vi "from string array.vi"(8 "error in (no error)":errorcluster, 9 "String Array":string[][](array[string]), 10 "version":string, 11 "module configuration in":refnum<class "tag select module configuration.lvclass">) -> (0 "error out":errorcluster, 3 "module configuration out":refnum<class "tag select module configuration.lvclass">)   [LabVIEW 2015, in "tag select module configuration.lvclass"]
uses:
  tag select module configuration.lvclass
  tag select configuration.ctl
  <vilib>/NI/Tag Bus/tag/Data Type.ctl
  <vilib>/NI/Tag Bus Module Framework/channel/TBM channel.lvclass
  <vilib>/NI/Tag Bus Module Framework/channel/channel classification.ctl
  tag select module configuration.lvclass/tag select module configuration.ctl
  Write tag select.vi
  <vilib>/NI/Tag Bus/tag/tag descriptor.lvclass
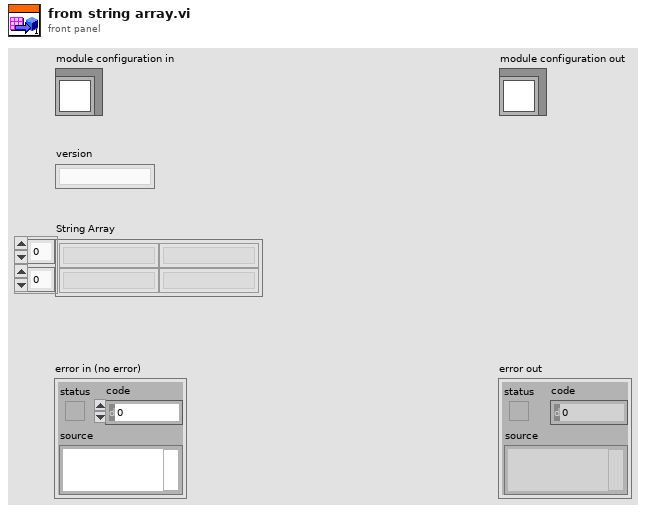
[diagram p1: front panel]
types:
  T1 = typedef "tag bus.lvlib/tag descriptor.lvclass/Data Type.ctl" = enum16{"Double", "Single", "I64", "I32", "I16", "I8", "U64", "U32", "U16", "U8", "Boolean", "String", "Array of Double", "Array of Single", "Array of I64", "Array of I32", "Array of I16", "Array of I8", "Array of U64", "Array of U32", "Array of U16", "Array of U8", "Array of Boolean", "Array of String"}
  T2 = typedef "TBM channel.lvclass/channel classification.ctl" = enum16{"input data", "output data", "processing parameter", "processing result"}
  T3 = typedef "tag select module configuration.lvclass/tag select configuration.ctl" = cluster{"tag select name":string, "data type":T1, "output":refnum<class "TBM channel.lvclass">, "select":refnum<class "TBM channel.lvclass">, "input channels":refnum<class "TBM channel.lvclass">[]}
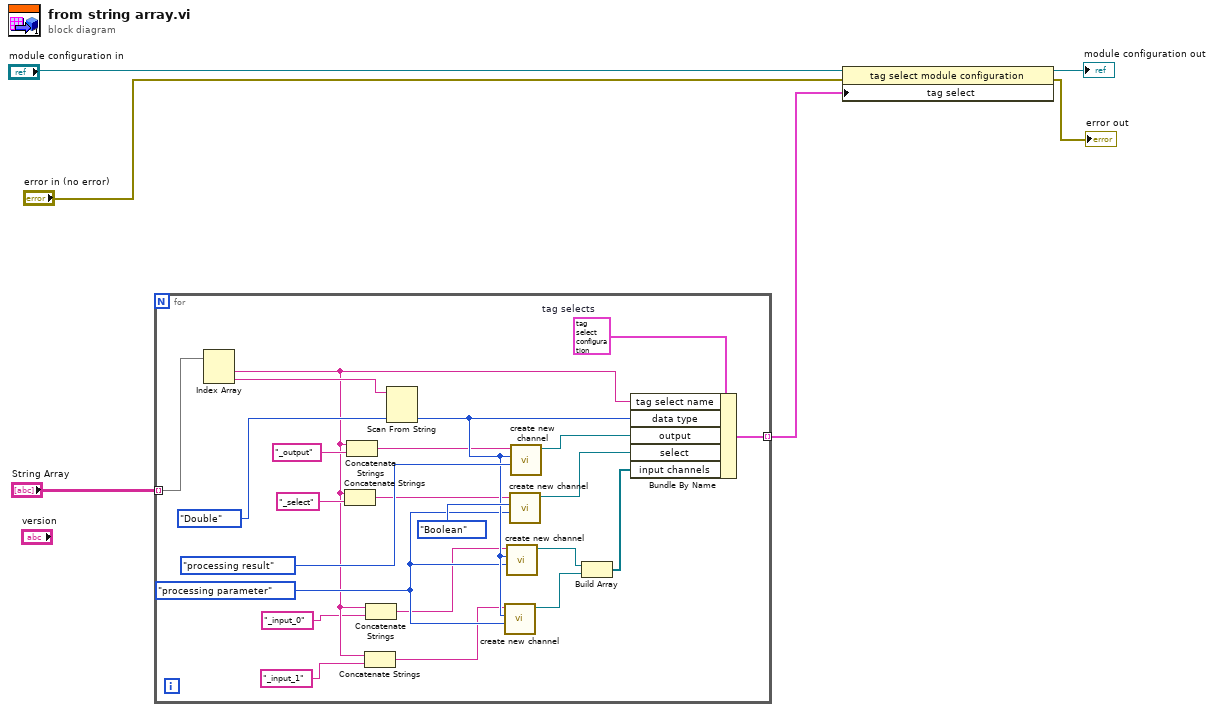
[diagram p0: block diagram]
diagram:
  n1 = for {
    tunnel: "String Array" -> [w28] mode=indexing
    tunnel: [w17] -> w1 mode=indexing
    w16 = channel_classification."processing parameter" ("channel classification")
    w29 = T3 {"tag select name"="", "data type"=enum."Double", "output"=refnum, "select"=refnum, "input channels"=[]}  # tag selects
    n2 = Index Array "Index Array"(array=w28) -> (element #1=w9:string, element #2=w27:string)  [unwired: 2 in]
    n3 = Concatenate Strings(w9, "_select" ("string")) -> (w13:string)
    n4 = Concatenate Strings(w9, "_output" ("string")) -> (w14:string)
    n5 = Concatenate Strings(w9, "_input_1" ("string")) -> (w10:string)
    n6 = Concatenate Strings(w9, "_input_0" ("string")) -> (w11:string)
    n7 = Scan From String(input string=w27, default 1=Data_Type."Double" ("data type")) -> (output 1=w21:T1)  [unwired: 3 in, 3 out]
    n8 = call <vilib>:"create new channel.vi"("channel classification"=w16, "data type"=w21, "channel name"=w10) -> ("channel"=w20:refnum<class "TBM channel.lvclass">)  [unwired: 8 in]
    n9 = call <vilib>:"create new channel.vi"("channel classification"=w16, "data type"=w21, "channel name"=w11) -> ("channel"=w19:refnum<class "TBM channel.lvclass">)  [unwired: 8 in]
    n10 = call <vilib>:"create new channel.vi"("channel classification"=w16, "data type"=Data_Type."Boolean", "channel name"=w13) -> ("channel"=w23:refnum<class "TBM channel.lvclass">)  [unwired: 8 in]
    n11 = call <vilib>:"create new channel.vi"("channel classification"=channel_classification."processing result", "data type"=w21, "channel name"=w14) -> ("channel"=w25:refnum<class "TBM channel.lvclass">)  [unwired: 8 in]
    n12 = Build Array(w19, w20) -> (w18:refnum<class "TBM channel.lvclass">[])
    n13 = Bundle By Name(cluster=w29, "tag select name"=w9, "data type"=w21, "output"=w25, "select"=w23, "input channels"=w18) -> (w17:T3)
  }
  n14 = property class="tag select module configuration"(reference="module configuration in", error in="error in (no error)", "tag select"=w1) -> (reference out=→"module configuration out":refnum<class "tag select module configuration.lvclass">, error out=→"error out":errorcluster)
